vi "labview_pra.vi"() -> ()   [LabVIEW 2017]
uses:
  <vilib>/addons/control/pid/pid.llb/PID (DBL).vi
  <vilib>/addons/control/pid/NI_PID_pid.lvlib
panel:
  out "结果":dbl
  in  "输入2":dbl
  in  "输入1":dbl
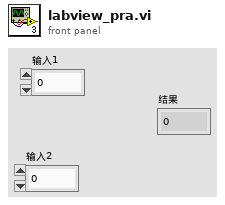
[diagram p1: front panel]
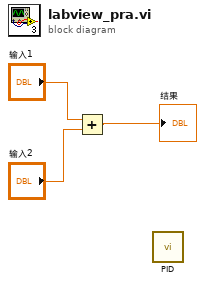
[diagram p0: block diagram]
diagram:
  n1 = Add(x="输入1", y="输入2") -> (x+y=→"结果":dbl)
  n2 = call-poly <vilib>:"PID.vi"() -> ()  [unwired: 10 in, 2 out]
